vi "Raw OutIn.vi"(7 "# of bytes to read in":i32=2, 8 "error in":errorcluster, 10 "Raw Out":u8[](array[numeric])=[8, 8] format="%.0x", 11 "Handle In":i32) -> (0 "error out":errorcluster, 2 "Raw In":u8[](array[numeric]) format="%.0x", 3 "Handle Out":i32, 5 "# of bytes read":i32)   [LabVIEW 2021]
panel:
  out "# of bytes written":i32
  # "This VI does the checksum check."
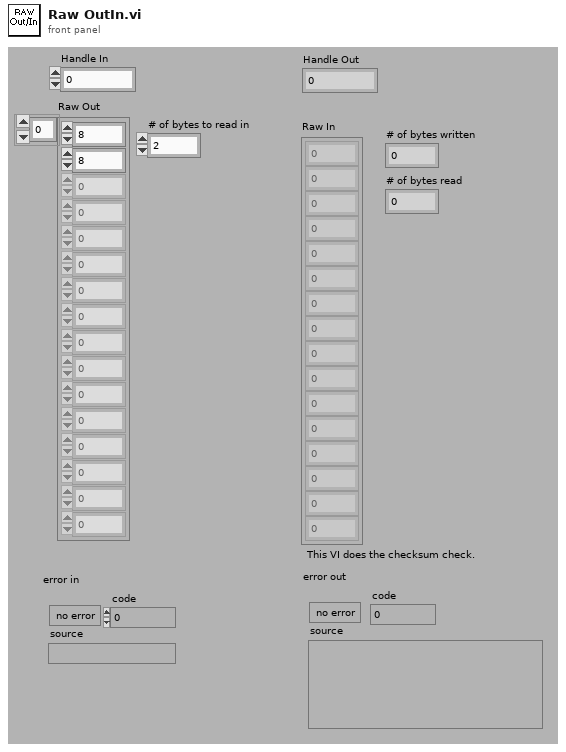
[diagram p1: front panel]
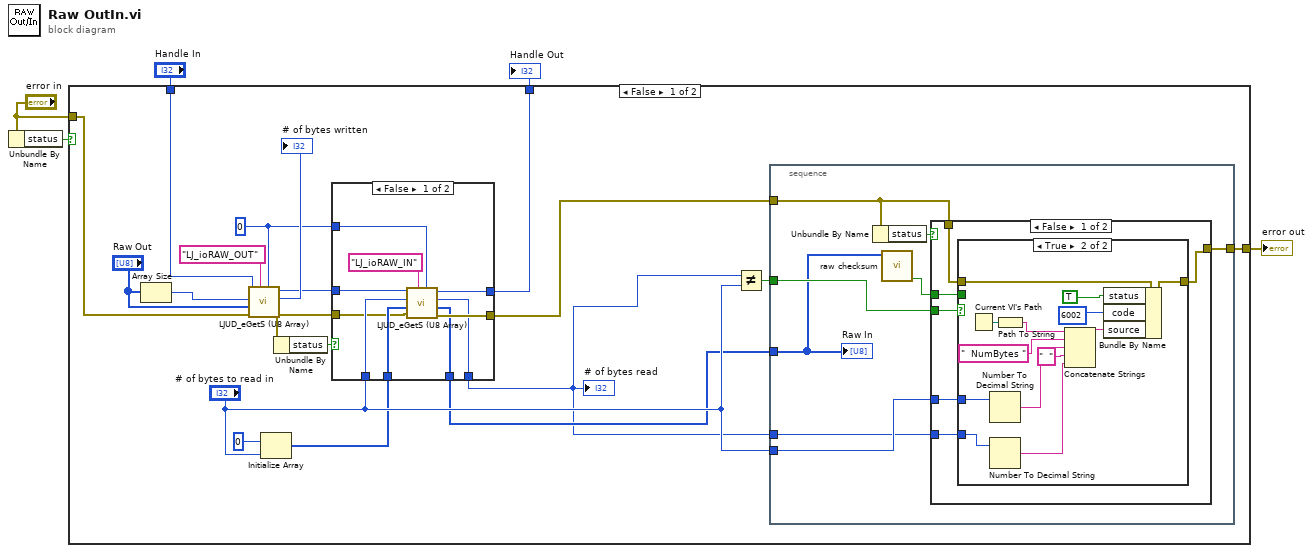
[diagram p0: block diagram]
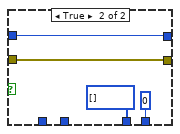
[diagram p2: hidden frame]
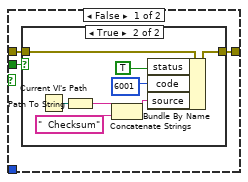
[diagram p3: hidden frame]
diagram:
  n1 = Unbundle By Name("error in") -> ("status"=w3:bool)
  n2 = case shown="False" w3 {
    tunnel: [w23 w80] -> w5
    tunnel: "error in" -> [w10 w80]
    tunnel: "Handle In" -> [w7 w79]
    tunnel: [w6 w79] -> w1
    frame False {
      w17 = 0 ("Channel")
      n3 = Array Size(array="Raw Out") -> (size(s)=w20:i32)
      n4 = call "LJUD_eGetS (U8 Array).vi"("Channel"=w17, "IOType"="LJ_ioRAW_OUT", "error in"=w10, "U8 Array Write"="Raw Out", "Value"=w20, "Handle In"=w7) -> ("error out"=w9:errorcluster, "Value"=→"# of bytes written":i32, "Handle Out"=w18:i32)  [unwired: 2 in, 1 out]
      n5 = Initialize Array(u8 0 ("Element Data"), "# of bytes to read in") -> (w15:u8[])
      n6 = Unbundle By Name(w9) -> ("status"=w8:bool)
      n7 = case shown="False" w8 {
        tunnel: [w34 w35] -> w12
        tunnel: w18 -> [w33 w38]
        tunnel: [w32 w38] -> w6
        tunnel: w17 -> [w31 _]
        tunnel: "# of bytes to read in" -> [w30 _]
        tunnel: w15 -> [w29 _]
        tunnel: [w28 u8[] [] ("U8 Array Read")] -> w14
        tunnel: [w27 0 ("# Elements Read")] -> w13
        tunnel: w9 -> [w25 w35]
        frame False {
          n8 = call "LJUD_eGetS (U8 Array).vi"("Channel"=w31, "IOType"="LJ_ioRAW_IN", "error in"=w25, "U8 Array Write"=w29, "Value"=w30, "Handle In"=w33) -> ("error out"=w34:errorcluster, "U8 Array Read"=w28:u8[], "Value"=w27:i32, "Handle Out"=w32:i32)  [unwired: 2 in]
        }
        frame True {
        }
      }
      "# of bytes read" <- w13
      n9 = Not Equal?(x=w13, y="# of bytes to read in") -> (x != y?=w22:bool)
      n10 = stacked-sequence {
        tunnel: w12 -> [w40]
        tunnel: [w46] -> w23
        tunnel: w22 -> [w44]
        tunnel: w14 -> [w43]
        tunnel: "# of bytes to read in" -> [w42]
        tunnel: w13 -> [w41]
        frame #0 {
          n11 = Unbundle By Name(w40) -> ("status"=w39:bool)
          n12 = call "raw checksum.vi"("Array"=w43) -> ("Checksum Error"=w45:bool)  [unwired: 3 in, 7 out]
          n13 = case shown="False" w39 {
            tunnel: [w52 w78] -> w46
            tunnel: w45 -> [w51 _]
            tunnel: w44 -> [w50 _]
            tunnel: w42 -> [w49 _]
            tunnel: w41 -> [w48 _]
            tunnel: w40 -> [w47 w78]
            frame False {
              n14 = case shown="True" w50 {
                tunnel: w47 -> [w55 w71]
                tunnel: [w54 w70] -> w52
                tunnel: w51 -> [w53 _]
                tunnel: w49 -> [_ w69]
                tunnel: w48 -> [_ w68]
                frame False {
                  n15 = case shown="True" w53 {
                    tunnel: w55 -> [w56 w58]
                    tunnel: [w56 w57] -> w54
                    frame False {
                    }
                    frame True {
                      n16 = Current VI's Path() -> (path=w61:path)
                      n17 = Path To String(path=w61) -> (string=w62:string)
                      n18 = Concatenate Strings(w62, "  Checksum" ("Substring")) -> (w63:string)
                      n19 = Bundle By Name(cluster=w58, "status"=TRUE, "code"=u32 6001 ("y"), "source"=w63) -> (w57:errorcluster)
                    }
                  }
                }
                frame True {
                  n20 = Current VI's Path() -> (path=w74:path)
                  n21 = Number To Decimal String(number=w69) -> (decimal integer string=w67:string)  [unwired: 1 in]
                  n22 = Number To Decimal String(number=w68) -> (decimal integer string=w65:string)  [unwired: 1 in]
                  n23 = Path To String(path=w74) -> (string=w75:string)
                  n24 = Concatenate Strings(w75, "  NumBytes " ("Substring"), w67, "  " ("Substring"), w65) -> (w76:string)
                  n25 = Bundle By Name(cluster=w71, "status"=TRUE, "code"=u32 6002 ("y"), "source"=w76) -> (w70:errorcluster)
                }
              }
            }
            frame True {
            }
          }
          "Raw In" <- w43
        }
      }
    }
    frame True {
    }
  }
  "error out" <- w5
  "Handle Out" <- w1
